vi "calibrated_to_raw.vi"   [LabVIEW 2015, in "lv-calibration.lvlib"]
uses:
  lv-calibration.lvlib
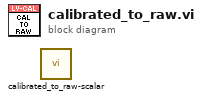
[diagram p0: block diagram]
diagram:
  n1 = call "calibrated_to_raw-scalar.vi"() -> ()  [unwired: 10 in, 2 out]
